vi "LAB1_pt2_ex2.vi"() -> ()   [LabVIEW 2015]
doc: "This example demonstrates how to read N channels of analog input from a LINX device."
uses:
  <vilib>/MakerHub/LINX/Public/Peripherals/PWM/PWM Set Duty Cycle 1 Chan.vi
  <vilib>/MakerHub/LINX/Public/Peripherals/Digital/Digital Write 1 Chan.vi
  <vilib>/MakerHub/LINX/Public/Peripherals/Digital/Digital Write N Chans.vi
  <vilib>/MakerHub/LINX/Private/Local IO/LinxDigitalWrite.vi
  <vilib>/MakerHub/LINX/Public/Utilities/Check Channel.vi
  <vilib>/MakerHub/LINX/Public/Utilities/Open Serial.vi
  <vilib>/MakerHub/LINX/Public/Peripherals/PWM/PWM Set Duty Cycle N Chans.vi
  <vilib>/MakerHub/LINX/Private/Utilties/Generate Error.vi
  <vilib>/MakerHub/LINX/LMH-LINX.lvlib
panel:
  in  "Thermometer":dbl(slide) scale=0.0..100.0
  in  "Stop Button 2":bool
  in  "T_Min":dbl
  out "Loop Rate (Hz)":u32
  out "Led Min":bool
  in  "Serial Port 2":refnum<visa-resource-name>
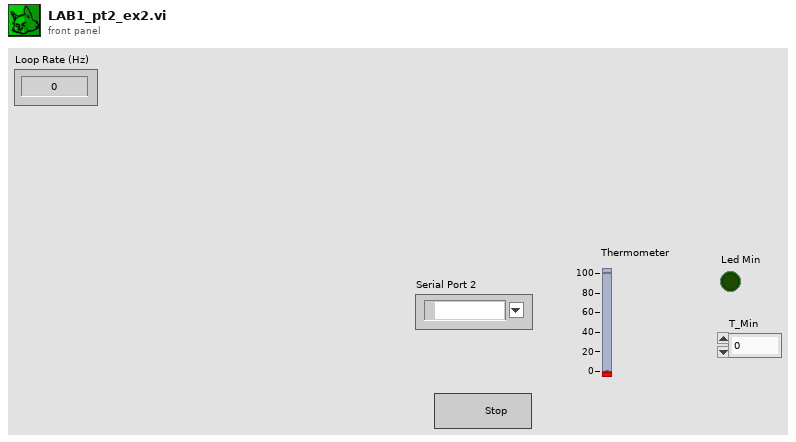
[diagram p1: front panel]
types:
  T1 = typedef "LMH-LINX.lvlib/LINX Ref.ctl" = cluster{"IO":T2, "Interface":T3, "LINX Device Config":T4}
  T2 = typedef "LMH-LINX.lvlib/Platform.ctl" = enum16{"Remote", "Local"}
  T3 = typedef "LMH-LINX.lvlib/Interface.ctl" = enum16{"Serial", "TCP"}
  T4 = typedef "LMH-LINX.lvlib/Device.lvlib/LINX Device Config.ctl" = cluster{"Interface":T3, "COM Port":refnum<visa-resource-name>, "TCP Configuration":T5, "Device Family":u8, "Device ID":u8, "Device Name":string, "TCP Ref":refnum<k5>, "Channels":T6}
  T5 = typedef "LMH-LINX.lvlib/Device.lvlib/TCP Config.ctl" = cluster{"IP Address":string, "Port":u16}
  T6 = typedef "LMH-LINX.lvlib/Channels.ctl" = cluster{"DI":u8[], "DO":u8[], "AI":u8[], "AO":u8[], "PWM":u8[], "QE":u8[], "UART":u8[], "I2C 2":u8[], "SPI":u8[], "CAN":u8[], "Servo":u8[], "AI Ref (V)":dbl, "AI Resolution (Bits)":u8, "AO Ref (V)":dbl, "AO Resolution (Bits)":u8}
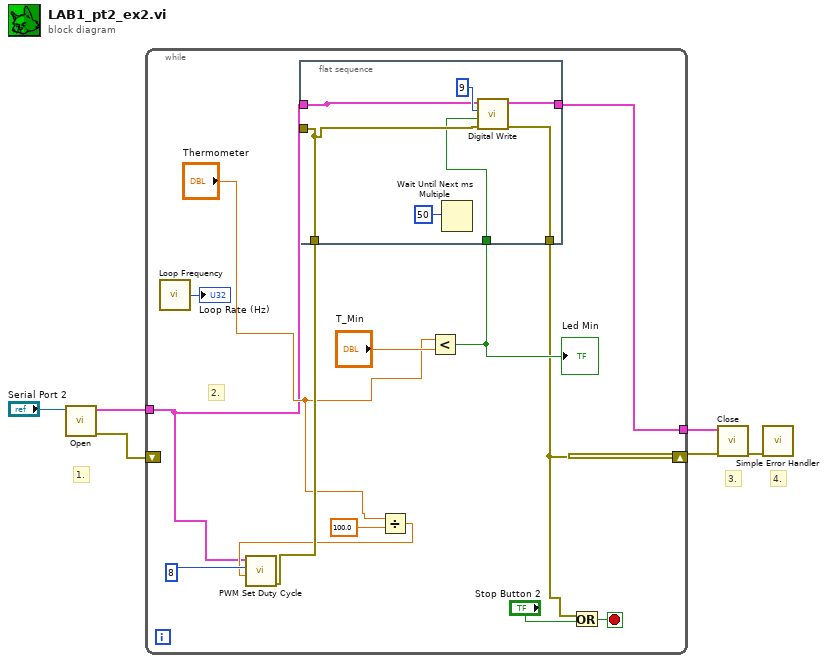
[diagram p0: block diagram]
diagram:
  # "4."
  # "3."
  # "1."
  n1 = call-poly <vilib>:"Open.vi"("Serial Port"="Serial Port 2") -> ("Error Out"=w5:errorcluster, "LINX Resource"=w6:T1)  [unwired: 8 in, 1 out]
  n2 = while {
    tunnel: w6 -> [w7]
    shift-right: [w13] -> w4
    shift-left: w5 -> [_]
    tunnel: [w15] -> w1
    stop <- w19 stop-if-true
    # "2."
    n3 = call <vilib>:"Loop Frequency.vi"() -> ("Loop Rate (Hz)"=→"Loop Rate (Hz)":u32)
    n4 = flat-sequence {
      tunnel: [w20] -> _
      tunnel: [w22] -> _
      tunnel: [w25] -> w15
      tunnel: w14 -> [w21]
      tunnel: [w23] -> w13
      tunnel: w12 -> [w22]
      tunnel: w7 -> [w20]
      frame #0 {
        n5 = Wait Until Next ms Multiple(millisecond multiple=u32 50) -> ()  [unwired: 1 out]
        n6 = call-poly <vilib>:"Digital Write.vi"("Error In"=w22, "Output Value"=w21, "DO Channel"=u8 9, "LINX Resource"=w20) -> ("Error Out"=w23:errorcluster, "LINX Resource"=w25:T1)  [unwired: 6 in]
      }
    }
    n7 = Divide(x="Thermometer", y=100.0 ("x")) -> (x/y=w8:dbl)
    n8 = call-poly <vilib>:"PWM Set Duty Cycle.vi"("Duty Cycle (0-1)"=w8, "PWM Channel"=8, "LINX Resource"=w7) -> ("Error Out"=w12:errorcluster)  [unwired: 7 in, 1 out]
    n9 = Less?(x="Thermometer", y="T_Min") -> (x < y?=w14:bool)
    "Led Min" <- w14
    n10 = Or(x=w13, y="Stop Button 2") -> (x .or. y?=w19:bool)
  }
  n11 = call <vilib>:"Close.vi"("Error In"=w4, "LINX Resource"=w1) -> ("Error Out"=w2:errorcluster)  [unwired: 9 in]
  n12 = call <vilib>:"Simple Error Handler.vi"("error in (no error)"=w2) -> ()  [unwired: 4 in, 5 out]
